vi "Clear XML Dependencies.vi"(8 "error in (no error)":errorcluster, 11 "Project XML Editor in":refnum<class "Project XML Editor.lvclass">) -> (0 "error out":errorcluster, 3 "Project XML Editor out":refnum<class "Project XML Editor.lvclass">)   [LabVIEW 2019, in "Project XML Editor.lvclass"]
uses:
  Project XML Editor.lvclass
  <vilib>/xml/Close Reference(Node).vi
  <resource>/objmgr/DOMUserDefRef.rc
  <vilib>/xml/NI_XML.lvlib
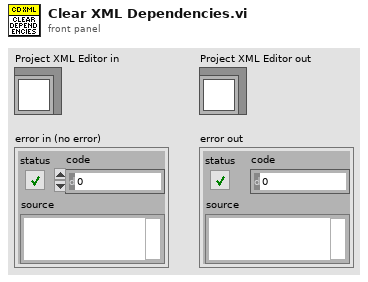
[diagram p1: front panel]
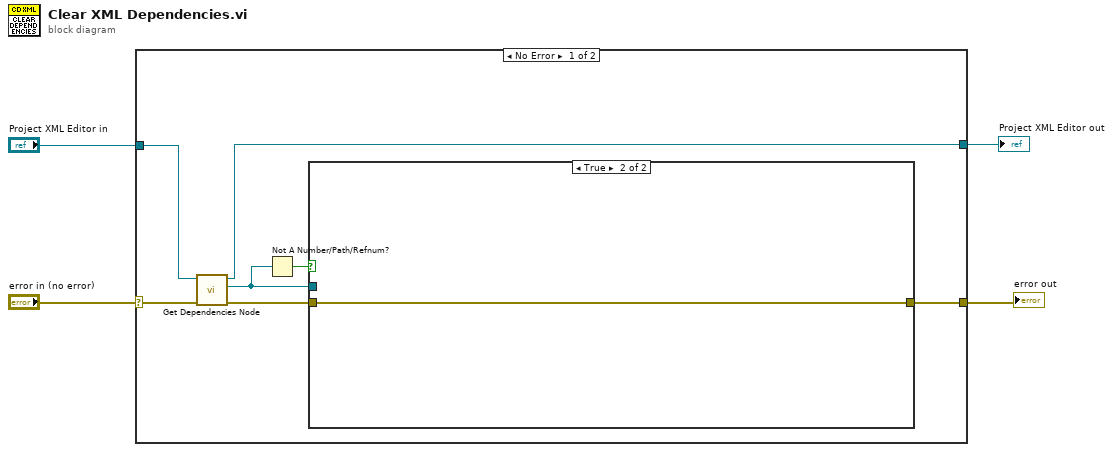
[diagram p0: block diagram]
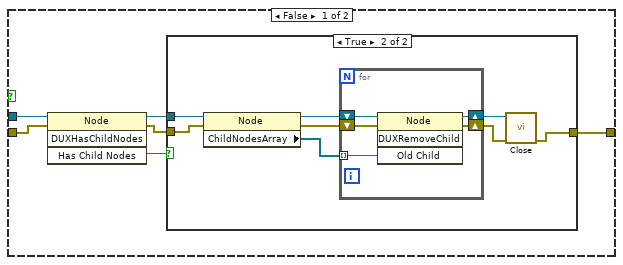
[diagram p2: hidden frame]
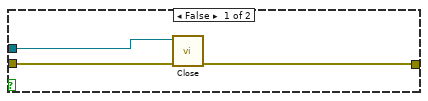
[diagram p3: hidden frame]
diagram:
  n1 = case shown="No Error" "error in (no error)" {
    selector: "error in (no error)" -> [w7 w35]
    tunnel: [w11 w35] -> w4
    tunnel: [w10 w36] -> w3
    tunnel: "Project XML Editor in" -> [w8 w36]
    frame No Error {
      n2 = call "Get Dependencies Node.vi"("error in (no error)"=w7, "Project XML Editor in"=w8) -> ("error out"=w9:errorcluster, "Dependencies out"=w6:refnum<k20>, "Project XML Editor out"=w10:refnum<class "Project XML Editor.lvclass">)  [unwired: 7 in]
      n3 = Not A Number/Path/Refnum?(number/path/refnum=w6) -> (NaN/Path/Refnum?=w5:bool)
      n4 = case shown="True" w5 {
        tunnel: [w17 w34] -> w11
        tunnel: w9 -> [w13 w34]
        tunnel: w6 -> [w12 _]
        frame False {
          n5 = invoke class="Node" method="DUXHasChildNodes"(reference=w12, error in=w13) -> (reference out=w16:refnum<k20>, error out=w15:errorcluster, "Has Child Nodes"=w14:bool)  [unwired: 2 in, 1 out]
          n6 = case shown="True" w14 {
            tunnel: w15 -> [w20 w28]
            tunnel: w16 -> [w19 w25]
            tunnel: [w18 w21] -> w17
            frame False {
              n7 = call-poly <vilib>:"Close.vi"("error in (no error)"=w20, "node"=w19) -> ("error out"=w18:errorcluster)  [unwired: 7 in]
            }
            frame True {
              n8 = property class="Node"(reference=w25, error in=w28) -> (reference out=w26:refnum<k20>, error out=w23:errorcluster, "ChildNodesArray"=w27:refnum<k20>[])
              n9 = for {
                tunnel: w27 -> [w29] mode=indexing
                shift-right: [w32] -> w24
                shift-left: w26 -> [w33]
                shift-right: [w30] -> w22
                shift-left: w23 -> [w31]
                n10 = invoke class="Node" method="DUXRemoveChild"(reference=w33, error in=w31, "Old Child"=w29) -> (reference out=w32:refnum<k20>, error out=w30:errorcluster)  [unwired: 1 in, 2 out]
              }
              n11 = call-poly <vilib>:"Close.vi"("error in (no error)"=w22, "node"=w24) -> ("error out"=w21:errorcluster)  [unwired: 7 in]
            }
          }
        }
        frame True {
        }
      }
    }
    frame Error {
    }
  }
  "error out" <- w4
  "Project XML Editor out" <- w3
